vi "RegisterForMessageSpecificType.vi"(8 "error in (no error)":errorcluster, 9 "Message Enqueuer":refnum<class "Message Enqueuer.lvclass">, 10 "Msg":refnum<class "MailBoxMessage.lvclass">, 11 "MailboxClientInterface in":refnum<class "MailboxClientInterface.lvclass">) -> (0 "error out":errorcluster, 3 "MailboxClientInterface out":refnum<class "MailboxClientInterface.lvclass">)   [LabVIEW 2020, in "MailboxManager.lvlib" / "MailboxClientInterface.lvclass"]
uses:
  MailboxClientInterface.lvclass
  MailboxManager/MailBoxMessage/MailBoxMessage.lvclass
  <vilib>/ActorFramework/Message Enqueuer/Message Enqueuer.lvclass
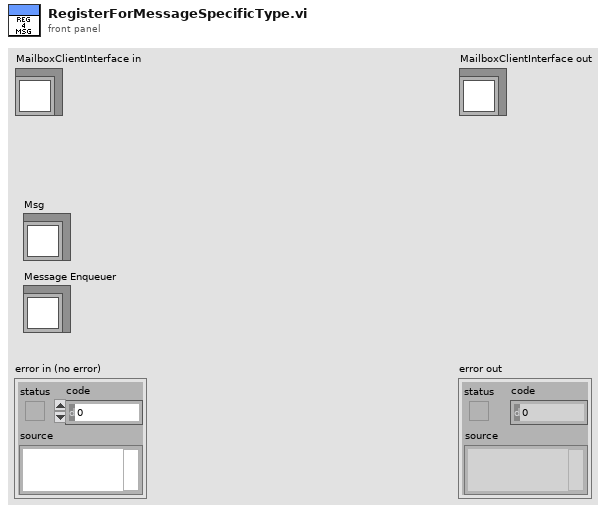
[diagram p1: front panel]
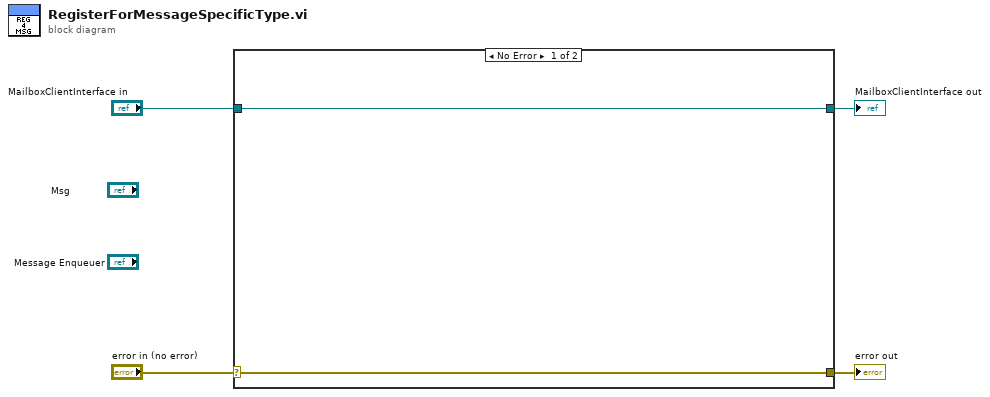
[diagram p0: block diagram]
diagram:
  n1 = case shown="No Error" "error in (no error)" {
    selector: "error in (no error)" -> [w5 w8]
    tunnel: [w5 w8] -> w3
    tunnel: [w6 w7] -> w1
    tunnel: "MailboxClientInterface in" -> [w6 w7]
    frame No Error {
    }
    frame Error {
    }
  }
  "error out" <- w3
  "MailboxClientInterface out" <- w1
